vi "time_lv2_unix.vi"(0 "unix_timestamp":dbl) -> (1 "lv_time":timestamp, 2 "lv_timestamp":dbl format="%.6f")   [LabVIEW 2018]
panel:
  # "Converts UNIX timestamp to LabView timestamp"
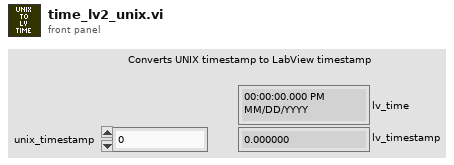
[diagram p1: front panel]
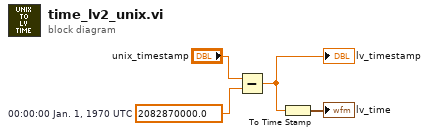
[diagram p0: block diagram]
diagram:
  w4 = 2082870000.0  # 00:00:00 Jan. 1, 1970 UTC
  n1 = Subtract(x="unix_timestamp", y=w4) -> (x-y=w2:dbl)
  "lv_timestamp" <- w2
  n2 = To Time Stamp(1:w2) -> (0:→"lv_time":timestamp)
